vi "GDSLvClass_GetClassName.vi"(0 "ViRef/Path,LvClassRef/Path":variant, 5 "error in (no error)":errorcluster) -> (14 "ClassRef":refnum<vi>, 15 "ClassName(without .lvclass)":string, 19 "error out":errorcluster)   [LabVIEW 2020]
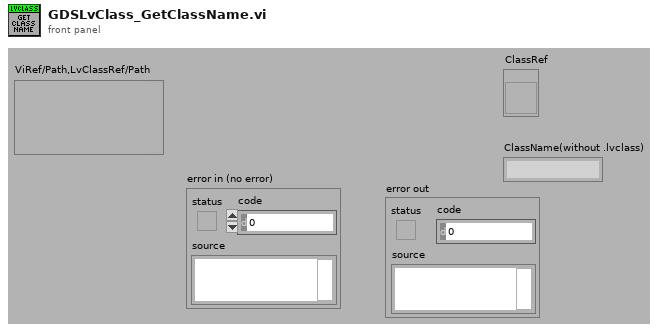
[diagram p1: front panel]
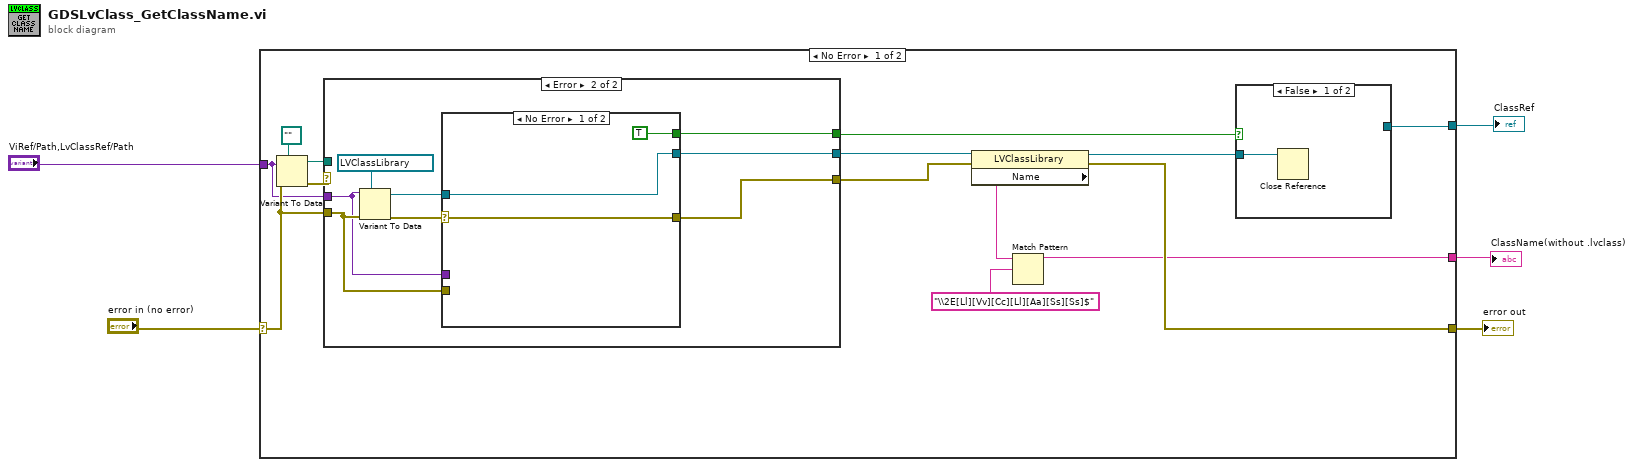
[diagram p0: block diagram]
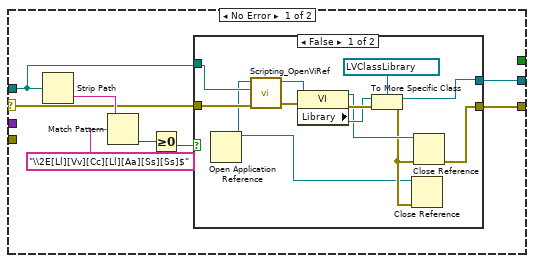
[diagram p3: hidden frame]
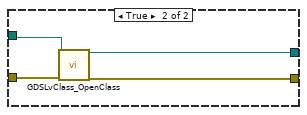
[diagram p4: hidden frame]
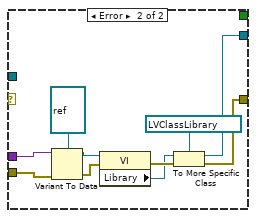
[diagram p5: hidden frame]
diagram:
  n1 = case shown="No Error" "error in (no error)" {
    selector: "error in (no error)" -> [w15 w67]
    tunnel: "ViRef/Path,LvClassRef/Path" -> [w14 _]
    tunnel: [w16 w67] -> w4
    tunnel: [w10 _] -> w2
    tunnel: [w7 _] -> w1
    frame No Error {
      n2 = Variant To Data(error in=w15, type=path "", Variant=w14) -> (data=w17:path, error out=w18:errorcluster)
      n3 = case shown="Error" w18 {
        selector: w18 -> [w25 _]
        tunnel: w17 -> [w26 _]
        tunnel: [w23 w48] -> w6
        tunnel: [w22 w49] -> w13
        tunnel: w15 -> [_ w52]
        tunnel: w14 -> [_ w47]
        tunnel: [_ w46] -> w12
        frame No Error {
          n4 = Strip Path(path=w26) -> (name=w28:string)  [unwired: 1 out]
          n5 = Match Pattern(string=w28, regular expression="\\2E[Ll][Vv][Cc][Ll][Aa][Ss][Ss]$") -> (offset past match=w27:i32)  [unwired: 1 in, 3 out]
          n6 = Greater Or Equal To 0?(x=w27) -> (x >= 0?=w24:bool)
          n7 = case shown="False" w24 {
            tunnel: w26 -> [w40 w45]
            tunnel: w25 -> [w41 w44]
            tunnel: [w32 w43] -> w23
            tunnel: [w34 w42] -> w22
            frame False {
              n8 = Open Application Reference() -> (3:w30:refnum<vi>)  [unwired: 4 in, 1 out]
              n9 = call "Scripting_OpenViRef.vi"("error in"=w41, "ViPath/ViName/Viref"=w40, "AppRef"=w30) -> ("error out"=w39:errorcluster, "vi reference"=w38:refnum<vi>)  [unwired: 6 in, 1 out]
              n10 = property class="VI"(reference=w38, error in=w39) -> (reference out=w33:refnum<vi>, error out=w37:errorcluster, "Library"=w36:refnum<vi>)
              n11 = To More Specific Class(target class=refnum<vi> refnum ("LVClass.Open"), reference=w36, error in=w37) -> (specific class reference=w34:refnum<vi>, error out=w31:errorcluster)
              n12 = Close Reference(reference=w30, error in (no error)=w31) -> ()  [unwired: 1 out]
              n13 = Close Reference(reference=w33, error in (no error)=w31) -> (error out=w32:errorcluster)
            }
            frame True {
              n14 = call "GDSLvClass_OpenClass.vi"("ClassToOpen"=w45, "error in (no error)"=w44) -> ("LVClass.Open"=w42:refnum<vi>, "error out"=w43:errorcluster)  [unwired: 16 in]
            }
          }
        }
        frame Error {
          n15 = Variant To Data(error in=w52, type=refnum<vi> refnum ("LVClass.Open"), Variant=w47) -> (data=w50:refnum<vi>, error out=w51:errorcluster)
          n16 = case shown="No Error" w51 {
            selector: w51 -> [w55 _]
            tunnel: w52 -> [_ w65]
            tunnel: w50 -> [w56 _]
            tunnel: [w56 w58] -> w49
            tunnel: [w55 w57] -> w48
            tunnel: w47 -> [_ w64]
            tunnel: [TRUE _] -> w46
            frame No Error {
            }
            frame Error {
              n17 = Variant To Data(error in=w65, type=refnum<vi> refnum ("vi reference"), Variant=w64) -> (data=w59:refnum<vi>, error out=w60:errorcluster)
              n18 = property class="VI"(reference=w59, error in=w60) -> (error out=w63:errorcluster, "Library"=w62:refnum<vi>)  [unwired: 1 out]
              n19 = To More Specific Class(target class=refnum<vi> refnum ("LVClass.Open"), reference=w62, error in=w63) -> (specific class reference=w58:refnum<vi>, error out=w57:errorcluster)
            }
          }
        }
      }
      n20 = property class="LVClassLibrary"(reference=w13, error in=w6) -> (reference out=w11:refnum<vi>, error out=w16:errorcluster, "Name"=w9:string)
      n21 = Match Pattern(string=w9, regular expression="\\2E[Ll][Vv][Cc][Ll][Aa][Ss][Ss]$") -> (before substring=w7:string)  [unwired: 1 in, 3 out]
      n22 = case shown="False" w12 {
        tunnel: w11 -> [w20 w21]
        tunnel: [_ w21] -> w10
        frame False {
          n23 = Close Reference(reference=w20) -> ()  [unwired: 1 in, 1 out]
        }
        frame True {
        }
      }
    }
    frame Error {
    }
  }
  "ClassRef" <- w2
  "ClassName(without .lvclass)" <- w1
  "error out" <- w4
